vi "joe_johnson_state_store.vi"(10 "data_store_mode":enum16{"Set", "Get"}(ring), 11 "joe_johnson_state":T1=enum."down") -> (1 "New Data":bool, 2 "Initialized":bool, 3 "joe_johnson_state out":T1=enum."down")   [LabVIEW 2011]
uses:
  joe_johnson_state.ctl
  <vilib>/Rock Robotics/WPI/DriverStation/WPI_DriverStationCommDataCacheOp.ctl
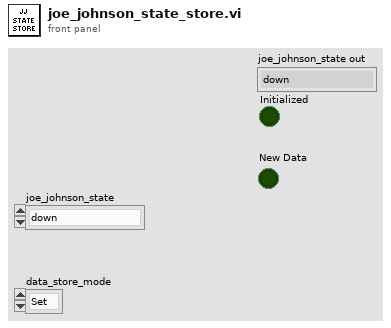
[diagram p1: front panel]
types:
  T1 = typedef "joe_johnson_state.ctl" = enum16{"fold", "down", "up", "ramp", "bridge_lift", "manual", "ramp_stay"}
  T2 = typedef "WPI_DriverStationCommDataCacheOp.ctl" = enum16{"Get", "Set", "Init"}
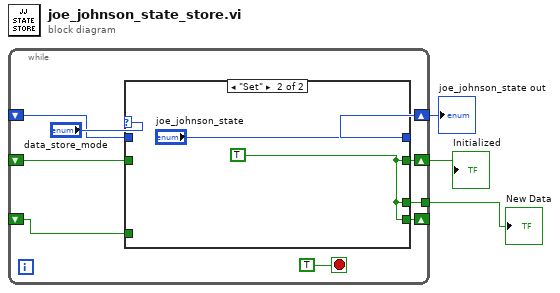
[diagram p0: block diagram]
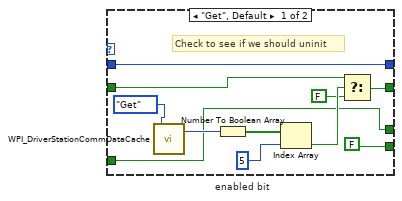
[diagram p2: hidden frame]
diagram:
  n1 = while {
    shift-right: [w10] -> w3
    shift-left: _ -> [w9]
    shift-right: [w8] -> w2
    shift-left: _ -> [w7]
    shift-right: [w5] -> _
    shift-left: _ -> [w4]
    tunnel: [w6] -> w1
    stop <- TRUE stop-if-true
    n2 = case shown="\"Set\"" "data_store_mode" {
      tunnel: [w23 "joe_johnson_state"] -> w10
      tunnel: w9 -> [w23 _]
      tunnel: [w16 w24] -> w8
      tunnel: w7 -> [w17 _]
      tunnel: [w14 w24] -> w6
      tunnel: [FALSE ("f") w24] -> w5
      tunnel: w4 -> [w14 _]
      frame "Get", Default {
        w21 = 5  # enabled bit
        # "Check to see if we should uninit"
        n3 = call <vilib>:"WPI_DriverStationCommDataCache.vi"("CommDataCacheOp"=WPI_DriverStationCommDataCacheOp."Get") -> ("ControlBit out"=w19:u8)  [unwired: 18 out]
        n4 = Number To Boolean Array(number=w19) -> (Boolean array=w20:bool[])
        n5 = Index Array(array=w20, index=w21) -> (element=w18:bool)
        n6 = Select(t=w17, s=w18, f=FALSE) -> (s? t:f=w16:bool)
      }
      frame "Set" {
        w24 = TRUE
      }
    }
  }
  "joe_johnson_state out" <- w3
  "Initialized" <- w2
  "New Data" <- w1
